vi "App - analyze RUS V6.vi"() -> ()   [LabVIEW 2018] (continued)
"z(0)"=0.0+0.0i, "radius"=0.0}}, "timestamp(min)"=2284.75, "timestamp"=timestamp(3493864906 s since 1904-01-01), "Magn Field(T)"=0.0}, {"temperature"=14.449, "lorentzian"={"A (VHz)"=0.0, "f (Hz)"=0.0, "G (Hz)"=0.0, "phi(rad)"=0.0, "Q"=0.0, "Norm  Ampl"=0.0, "bg (V)"=0.0+0.0i, "4corners"={"z (-pi/2)"=0.0+0.0i, "z(inf)"=0.0+0.0i, "z (pi/2)"=0.0+0.0i, "z center"=0.0+0.0i, "z(0)"=0.0+0.0i, "radius"=0.0}}, "timestamp(min)"=2286.083333335817, "timestamp"=timestamp(3493864986 s since 1904-01-01), "Magn Field(T)"=0.0}, {"temperature"=14.451, "lorentzian"={"A (VHz)"=0.0, "f (Hz)"=0.0, "G (Hz)"=0.0, "phi(rad)"=0.0, "Q"=0.0, "Norm  Ampl"=0.0, "bg (V)"=0.0+0.0i, "4corners"={"z (-pi/2)"=0.0+0.0i, "z(inf)"=0.0+0.0i, "z (pi/2)"=0.0+0.0i, "z center"=0.0+0.0i, "z(0)"=0.0+0.0i, "radius"=0.0}}, "timestamp(min)"=2287.39999999851, "timestamp"=timestamp(3493865065 s since 1904-01-01), "Magn Field(T)"=0.0}, {"temperature"=14.449, "lorentzian"={"A (VHz)"=0.0, "f (Hz)"=0.0, "G (Hz)"=0.0, "phi(rad)"=0.0, "Q"=0.0, "Norm  Ampl"=0.0, "bg (V)"=0.0+0.0i, "4corners"={"z (-pi/2)"=0.0+0.0i, "z(inf)"=0.0+0.0i, "z (pi/2)"=0.0+0.0i, "z center"=0.0+0.0i, "z(0)"=0.0+0.0i, "radius"=0.0}}, "timestamp(min)"=2288.7333333343267, "timestamp"=timestamp(3493865145 s since 1904-01-01), "Magn Field(T)"=0.0}, {"temperature"=14.445, "lorentzian"={"A (VHz)"=0.0, "f (Hz)"=0.0, "G (Hz)"=0.0, "phi(rad)"=0.0, "Q"=0.0, "Norm  Ampl"=0.0, "bg (V)"=0.0+0.0i, "4corners"={"z (-pi/2)"=0.0+0.0i, "z(inf)"=0.0+0.0i, "z (pi/2)"=0.0+0.0i, "z center"=0.0+0.0i, "z(0)"=0.0+0.0i, "radius"=0.0}}, "timestamp(min)"=2290.0500000044703, "timestamp"=timestamp(3493865224 s since 1904-01-01), "Magn Field(T)"=0.0}, {"temperature"=14.447, "lorentzian"={"A (VHz)"=0.0, "f (Hz)"=0.0, "G (Hz)"=0.0, "phi(rad)"=0.0, "Q"=0.0, "Norm  Ampl"=0.0, "bg (V)"=0.0+0.0i, "4corners"={"z (-pi/2)"=0.0+0.0i, "z(inf)"=0.0+0.0i, "z (pi/2)"=0.0+0.0i, "z center"=0.0+0.0i, "z(0)"=0.0+0.0i, "radius"=0.0}}, "timestamp(min)"=2291.3666666671634, "timestamp"=timestamp(3493865303 s since 1904-01-01), "Magn Field(T)"=0.0}, {"temperature"=14.443, "lorentzian"={"A (VHz)"=0.0, "f (Hz)"=0.0, "G (Hz)"=0.0, "phi(rad)"=0.0, "Q"=0.0, "Norm  Ampl"=0.0, "bg (V)"=0.0+0.0i, "4corners"={"z (-pi/2)"=0.0+0.0i, "z(inf)"=0.0+0.0i, "z (pi/2)"=0.0+0.0i, "z center"=0.0+0.0i, "z(0)"=0.0+0.0i, "radius"=0.0}}, "timestamp(min)"=2292.7000000029802, "timestamp"=timestamp(3493865383 s since 1904-01-01), "Magn Field(T)"=0.0}, {"temperature"=14.439, "lorentzian"={"A (VHz)"=0.0, "f (Hz)"=0.0, "G (Hz)"=0.0, "phi(rad)"=0.0, "Q"=0.0, "Norm  Ampl"=0.0, "bg (V)"=0.0+0.0i, "4corners"={"z (-pi/2)"=0.0+0.0i, "z(inf)"=0.0+0.0i, "z (pi/2)"=0.0+0.0i, "z center"=0.0+0.0i, "z(0)"=0.0+0.0i, "radius"=0.0}}, "timestamp(min)"=2294.0166666656733, "timestamp"=timestamp(3493865462 s since 1904-01-01), "Magn Field(T)"=0.0}, {"temperature"=14.439, "lorentzian"={"A (VHz)"=0.0, "f (Hz)"=0.0, "G (Hz)"=0.0, "phi(rad)"=0.0, "Q"=0.0, "Norm  Ampl"=0.0, "bg (V)"=0.0+0.0i, "4corners"={"z (-pi/2)"=0.0+0.0i, "z(inf)"=0.0+0.0i, "z (pi/2)"=0.0+0.0i, "z center"=0.0+0.0i, "z(0)"=0.0+0.0i, "radius"=0.0}}, "timestamp(min)"=2295.333333335817, "timestamp"=timestamp(3493865541 s since 1904-01-01), "Magn Field(T)"=0.0}, {"temperature"=14.439, "lorentzian"={"A (VHz)"=0.0, "f (Hz)"=0.0, "G (Hz)"=0.0, "phi(rad)"=0.0, "Q"=0.0, "Norm  Ampl"=0.0, "bg (V)"=0.0+0.0i, "4corners"={"z (-pi/2)"=0.0+0.0i, "z(inf)"=0.0+0.0i, "z (pi/2)"=0.0+0.0i, "z center"=0.0+0.0i, "z(0)"=0.0+0.0i, "radius"=0.0}}, "timestamp(min)"=2296.666666664183, "timestamp"=timestamp(3493865621 s since 1904-01-01), "Magn Field(T)"=0.0}, {"temperature"=14.439, "lorentzian"={"A (VHz)"=0.0, "f (Hz)"=0.0, "G (Hz)"=0.0, "phi(rad)"=0.0, "Q"=0.0, "Norm  Ampl"=0.0, "bg (V)"=0.0+0.0i, "4corners"={"z (-pi/2)"=0.0+0.0i, "z(inf)"=0.0+0.0i, "z (pi/2)"=0.0+0.0i, "z center"=0.0+0.0i, "z(0)"=0.0+0.0i, "radius"=0.0}}, "timestamp(min)"=2297.9833333343267, "timestamp"=timestamp(3493865700 s since 1904-01-01), "Magn Field(T)"=0.0}, {"temperature"=14.44, "lorentzian"={"A (VHz)"=0.0, "f (Hz)"=0.0, "G (Hz)"=0.0, "phi(rad)"=0.0, "Q"=0.0, "Norm  Ampl"=0.0, "bg (V)"=0.0+0.0i, "4corners"={"z (-pi/2)"=0.0+0.0i, "z(inf)"=0.0+0.0i, "z (pi/2)"=0.0+0.0i, "z center"=0.0+0.0i, "z(0)"=0.0+0.0i, "radius"=0.0}}, "timestamp(min)"=2299.3166666701436, "timestamp"=timestamp(3493865780 s since 1904-01-01), "Magn Field(T)"=0.0}, {"temperature"=14.433, "lorentzian"={"A (VHz)"=0.0, "f (Hz)"=0.0, "G (Hz)"=0.0, "phi(rad)"=0.0, "Q"=0.0, "Norm  Ampl"=0.0, "bg (V)"=0.0+0.0i, "4corners"={"z (-pi/2)"=0.0+0.0i, "z(inf)"=0.0+0.0i, "z (pi/2)"=0.0+0.0i, "z center"=0.0+0.0i, "z(0)"=0.0+0.0i, "radius"=0.0}}, "timestamp(min)"=2300.6333333328366, "timestamp"=timestamp(3493865859 s since 1904-01-01), "Magn Field(T)"=0.0}, {"temperature"=14.434, "lorentzian"={"A (VHz)"=0.0, "f (Hz)"=0.0, "G (Hz)"=0.0, "phi(rad)"=0.0, "Q"=0.0, "Norm  Ampl"=0.0, "bg (V)"=0.0+0.0i, "4corners"={"z (-pi/2)"=0.0+0.0i, "z(inf)"=0.0+0.0i, "z (pi/2)"=0.0+0.0i, "z center"=0.0+0.0i, "z(0)"=0.0+0.0i, "radius"=0.0}}, "timestamp(min)"=2301.9500000029802, "timestamp"=timestamp(3493865938 s since 1904-01-01), "Magn Field(T)"=0.0}, {"temperature"=14.43, "lorentzian"={"A (VHz)"=0.0, "f (Hz)"=0.0, "G (Hz)"=0.0, "phi(rad)"=0.0, "Q"=0.0, "Norm  Ampl"=0.0, "bg (V)"=0.0+0.0i, "4corners"={"z (-pi/2)"=0.0+0.0i, "z(inf)"=0.0+0.0i, "z (pi/2)"=0.0+0.0i, "z center"=0.0+0.0i, "z(0)"=0.0+0.0i, "radius"=0.0}}, "timestamp(min)"=2303.2833333313465, "timestamp"=timestamp(3493866018 s since 1904-01-01), "Magn Field(T)"=0.0}, {"temperature"=14.43, "lorentzian"={"A (VHz)"=0.0, "f (Hz)"=0.0, "G (Hz)"=0.0, "phi(rad)"=0.0, "Q"=0.0, "Norm  Ampl"=0.0, "bg (V)"=0.0+0.0i, "4corners"={"z (-pi/2)"=0.0+0.0i, "z(inf)"=0.0+0.0i, "z (pi/2)"=0.0+0.0i, "z center"=0.0+0.0i, "z(0)"=0.0+0.0i, "radius"=0.0}}, "timestamp(min)"=2304.60000000149, "timestamp"=timestamp(3493866097 s since 1904-01-01), "Magn Field(T)"=0.0}, {"temperature"=14.43, "lorentzian"={"A (VHz)"=0.0, "f (Hz)"=0.0, "G (Hz)"=0.0, "phi(rad)"=0.0, "Q"=0.0, "Norm  Ampl"=0.0, "bg (V)"=0.0+0.0i, "4corners"={"z (-pi/2)"=0.0+0.0i, "z(inf)"=0.0+0.0i, "z (pi/2)"=0.0+0.0i, "z center"=0.0+0.0i, "z(0)"=0.0+0.0i, "radius"=0.0}}, "timestamp(min)"=2305.933333337307, "timestamp"=timestamp(3493866177 s since 1904-01-01), "Magn Field(T)"=0.0}, {"temperature"=14.434, "lorentzian"={"A (VHz)"=0.0, "f (Hz)"=0.0, "G (Hz)"=0.0, "phi(rad)"=0.0, "Q"=0.0, "Norm  Ampl"=0.0, "bg (V)"=0.0+0.0i, "4corners"={"z (-pi/2)"=0.0+0.0i, "z(inf)"=0.0+0.0i, "z (pi/2)"=0.0+0.0i, "z center"=0.0+0.0i, "z(0)"=0.0+0.0i, "radius"=0.0}}, "timestamp(min)"=2307.25, "timestamp"=timestamp(3493866256 s since 1904-01-01), "Magn Field(T)"=0.0}, {"temperature"=14.434, "lorentzian"={"A (VHz)"=0.0, "f (Hz)"=0.0, "G (Hz)"=0.0, "phi(rad)"=0.0, "Q"=0.0, "Norm  Ampl"=0.0, "bg (V)"=0.0+0.0i, "4corners"={"z (-pi/2)"=0.0+0.0i, "z(inf)"=0.0+0.0i, "z (pi/2)"=0.0+0.0i, "z center"=0.0+0.0i, "z(0)"=0.0+0.0i, "radius"=0.0}}, "timestamp(min)"=2308.5666666701436, "timestamp"=timestamp(3493866335 s since 1904-01-01), "Magn Field(T)"=0.0}, {"temperature"=14.431, "lorentzian"={"A (VHz)"=0.0, "f (Hz)"=0.0, "G (Hz)"=0.0, "phi(rad)"=0.0, "Q"=0.0, "Norm  Ampl"=0.0, "bg (V)"=0.0+0.0i, "4corners"={"z (-pi/2)"=0.0+0.0i, "z(inf)"=0.0+0.0i, "z (pi/2)"=0.0+0.0i, "z center"=0.0+0.0i, "z(0)"=0.0+0.0i, "radius"=0.0}}, "timestamp(min)"=2309.89999999851, "timestamp"=timestamp(3493866415 s since 1904-01-01), "Magn Field(T)"=0.0}, {"temperature"=14.429, "lorentzian"={"A (VHz)"=0.0, "f (Hz)"=0.0, "G (Hz)"=0.0, "phi(rad)"=0.0, "Q"=0.0, "Norm  Ampl"=0.0, "bg (V)"=0.0+0.0i, "4corners"={"z (-pi/2)"=0.0+0.0i, "z(inf)"=0.0+0.0i, "z (pi/2)"=0.0+0.0i, "z center"=0.0+0.0i, "z(0)"=0.0+0.0i, "radius"=0.0}}, "timestamp(min)"=2311.2166666686535, "timestamp"=timestamp(3493866494 s since 1904-01-01), "Magn Field(T)"=0.0}, {"temperature"=14.426, "lorentzian"={"A (VHz)"=0.0, "f (Hz)"=0.0, "G (Hz)"=0.0, "phi(rad)"=0.0, "Q"=0.0, "Norm  Ampl"=0.0, "bg (V)"=0.0+0.0i, "4corners"={"z (-pi/2)"=0.0+0.0i, "z(inf)"=0.0+0.0i, "z (pi/2)"=0.0+0.0i, "z center"=0.0+0.0i, "z(0)"=0.0+0.0i, "radius"=0.0}}, "timestamp(min)"=2312.5333333313465, "timestamp"=timestamp(3493866573 s since 1904-01-01), "Magn Field(T)"=0.0}, {"temperature"=14.429, "lorentzian"={"A (VHz)"=0.0, "f (Hz)"=0.0, "G (Hz)"=0.0, "phi(rad)"=0.0, "Q"=0.0, "Norm  Ampl"=0.0, "bg (V)"=0.0+0.0i, "4corners"={"z (-pi/2)"=0.0+0.0i, "z(inf)"=0.0+0.0i, "z (pi/2)"=0.0+0.0i, "z center"=0.0+0.0i, "z(0)"=0.0+0.0i, "radius"=0.0}}, "timestamp(min)"=2313.8666666671634, "timestamp"=timestamp(3493866653 s since 1904-01-01), "Magn Field(T)"=0.0}, {"temperature"=14.429, "lorentzian"={"A (VHz)"=0.0, "f (Hz)"=0.0, "G (Hz)"=0.0, "phi(rad)"=0.0, "Q"=0.0, "Norm  Ampl"=0.0, "bg (V)"=0.0+0.0i, "4corners"={"z (-pi/2)"=0.0+0.0i, "z(inf)"=0.0+0.0i, "z (pi/2)"=0.0+0.0i, "z center"=0.0+0.0i, "z(0)"=0.0+0.0i, "radius"=0.0}}, "timestamp(min)"=2315.183333337307, "timestamp"=timestamp(3493866732 s since 1904-01-01), "Magn Field(T)"=0.0}, {"temperature"=14.425, "lorentzian"={"A (VHz)"=0.0, "f (Hz)"=0.0, "G (Hz)"=0.0, "phi(rad)"=0.0, "Q"=0.0, "Norm  Ampl"=0.0, "bg (V)"=0.0+0.0i, "4corners"={"z (-pi/2)"=0.0+0.0i, "z(inf)"=0.0+0.0i, "z (pi/2)"=0.0+0.0i, "z center"=0.0+0.0i, "z(0)"=0.0+0.0i, "radius"=0.0}}, "timestamp(min)"=2316.5166666656733, "timestamp"=timestamp(3493866812 s since 1904-01-01), "Magn Field(T)"=0.0}, {"temperature"=14.426, "lorentzian"={"A (VHz)"=0.0, "f (Hz)"=0.0, "G (Hz)"=0.0, "phi(rad)"=0.0, "Q"=0.0, "Norm  Ampl"=0.0, "bg (V)"=0.0+0.0i, "4corners"={"z (-pi/2)"=0.0+0.0i, "z(inf)"=0.0+0.0i, "z (pi/2)"=0.0+0.0i, "z center"=0.0+0.0i, "z(0)"=0.0+0.0i, "radius"=0.0}}, "timestamp(min)"=2317.833333335817, "timestamp"=timestamp(3493866891 s since 1904-01-01), "Magn Field(T)"=0.0}, {"temperature"=14.422, "lorentzian"={"A (VHz)"=0.0, "f (Hz)"=0.0, "G (Hz)"=0.0, "phi(rad)"=0.0, "Q"=0.0, "Norm  Ampl"=0.0, "bg (V)"=0.0+0.0i, "4corners"={"z (-pi/2)"=0.0+0.0i, "z(inf)"=0.0+0.0i, "z (pi/2)"=0.0+0.0i, "z center"=0.0+0.0i, "z(0)"=0.0+0.0i, "radius"=0.0}}, "timestamp(min)"=2319.14999999851, "timestamp"=timestamp(3493866970 s since 1904-01-01), "Magn Field(T)"=0.0}, {"temperature"=14.424, "lorentzian"={"A (VHz)"=0.0, "f (Hz)"=0.0, "G (Hz)"=0.0, "phi(rad)"=0.0, "Q"=0.0, "Norm  Ampl"=0.0, "bg (V)"=0.0+0.0i, "4corners"={"z (-pi/2)"=0.0+0.0i, "z(inf)"=0.0+0.0i, "z (pi/2)"=0.0+0.0i, "z center"=0.0+0.0i, "z(0)"=0.0+0.0i, "radius"=0.0}}, "timestamp(min)"=2320.4833333343267, "timestamp"=timestamp(3493867050 s since 1904-01-01), "Magn Field(T)"=0.0}, {"temperature"=14.421, "lorentzian"={"A (VHz)"=0.0, "f (Hz)"=0.0, "G (Hz)"=0.0, "phi(rad)"=0.0, "Q"=0.0, "Norm  Ampl"=0.0, "bg (V)"=0.0+0.0i, "4corners"={"z (-pi/2)"=0.0+0.0i, "z(inf)"=0.0+0.0i, "z (pi/2)"=0.0+0.0i, "z center"=0.0+0.0i, "z(0)"=0.0+0.0i, "radius"=0.0}}, "timestamp(min)"=2321.8000000044703, "timestamp"=timestamp(3493867129 s since 1904-01-01), "Magn Field(T)"=0.0}, {"temperature"=14.418, "lorentzian"={"A (VHz)"=0.0, "f (Hz)"=0.0, "G (Hz)"=0.0, "phi(rad)"=0.0, "Q"=0.0, "Norm  Ampl"=0.0, "bg (V)"=0.0+0.0i, "4corners"={"z (-pi/2)"=0.0+0.0i, "z(inf)"=0.0+0.0i, "z (pi/2)"=0.0+0.0i, "z center"=0.0+0.0i, "z(0)"=0.0+0.0i, "radius"=0.0}}, "timestamp(min)"=2323.1166666671634, "timestamp"=timestamp(3493867208 s since 1904-01-01), "Magn Field(T)"=0.0}, {"temperature"=14.417, "lorentzian"={"A (VHz)"=0.0, "f (Hz)"=0.0, "G (Hz)"=0.0, "phi(rad)"=0.0, "Q"=0.0, "Norm  Ampl"=0.0, "bg (V)"=0.0+0.0i, "4corners"={"z (-pi/2)"=0.0+0.0i, "z(inf)"=0.0+0.0i, "z (pi/2)"=0.0+0.0i, "z center"=0.0+0.0i, "z(0)"=0.0+0.0i, "radius"=0.0}}, "timestamp(min)"=2324.4500000029802, "timestamp"=timestamp(3493867288 s since 1904-01-01), "Magn Field(T)"=0.0}, {"temperature"=14.415, "lorentzian"={"A (VHz)"=0.0, "f (Hz)"=0.0, "G (Hz)"=0.0, "phi(rad)"=0.0, "Q"=0.0, "Norm  Ampl"=0.0, "bg (V)"=0.0+0.0i, "4corners"={"z (-pi/2)"=0.0+0.0i, "z(inf)"=0.0+0.0i, "z (pi/2)"=0.0+0.0i, "z center"=0.0+0.0i, "z(0)"=0.0+0.0i, "radius"=0.0}}, "timestamp(min)"=2325.7666666656733, "timestamp"=timestamp(3493867367 s since 1904-01-01), "Magn Field(T)"=0.0}, {"temperature"=14.413, "lorentzian"={"A (VHz)"=0.0, "f (Hz)"=0.0, "G (Hz)"=0.0, "phi(rad)"=0.0, "Q"=0.0, "Norm  Ampl"=0.0, "bg (V)"=0.0+0.0i, "4corners"={"z (-pi/2)"=0.0+0.0i, "z(inf)"=0.0+0.0i, "z (pi/2)"=0.0+0.0i, "z center"=0.0+0.0i, "z(0)"=0.0+0.0i, "radius"=0.0}}, "timestamp(min)"=2327.10000000149, "timestamp"=timestamp(3493867447 s since 1904-01-01), "Magn Field(T)"=0.0}, {"temperature"=14.414, "lorentzian"={"A (VHz)"=0.0, "f (Hz)"=0.0, "G (Hz)"=0.0, "phi(rad)"=0.0, "Q"=0.0, "Norm  Ampl"=0.0, "bg (V)"=0.0+0.0i, "4corners"={"z (-pi/2)"=0.0+0.0i, "z(inf)"=0.0+0.0i, "z (pi/2)"=0.0+0.0i, "z center"=0.0+0.0i, "z(0)"=0.0+0.0i, "radius"=0.0}}, "timestamp(min)"=2328.416666664183, "timestamp"=timestamp(3493867526 s since 1904-01-01), "Magn Field(T)"=0.0}, {"temperature"=14.412, "lorentzian"={"A (VHz)"=0.0, "f (Hz)"=0.0, "G (Hz)"=0.0, "phi(rad)"=0.0, "Q"=0.0, "Norm  Ampl"=0.0, "bg (V)"=0.0+0.0i, "4corners"={"z (-pi/2)"=0.0+0.0i, "z(inf)"=0.0+0.0i, "z (pi/2)"=0.0+0.0i, "z center"=0.0+0.0i, "z(0)"=0.0+0.0i, "radius"=0.0}}, "timestamp(min)"=2329.7333333343267, "timestamp"=timestamp(3493867605 s since 1904-01-01), "Magn Field(T)"=0.0}, {"temperature"=14.418, "lorentzian"={"A (VHz)"=0.0, "f (Hz)"=0.0, "G (Hz)"=0.0, "phi(rad)"=0.0, "Q"=0.0, "Norm  Ampl"=0.0, "bg (V)"=0.0+0.0i, "4corners"={"z (-pi/2)"=0.0+0.0i, "z(inf)"=0.0+0.0i, "z (pi/2)"=0.0+0.0i, "z center"=0.0+0.0i, "z(0)"=0.0+0.0i, "radius"=0.0}}, "timestamp(min)"=2331.0666666701436, "timestamp"=timestamp(3493867685 s since 1904-01-01), "Magn Field(T)"=0.0}, {"temperature"=14.417, "lorentzian"={"A (VHz)"=0.0, "f (Hz)"=0.0, "G (Hz)"=0.0, "phi(rad)"=0.0, "Q"=0.0, "Norm  Ampl"=0.0, "bg (V)"=0.0+0.0i, "4corners"={"z (-pi/2)"=0.0+0.0i, "z(inf)"=0.0+0.0i, "z (pi/2)"=0.0+0.0i, "z center"=0.0+0.0i, "z(0)"=0.0+0.0i, "radius"=0.0}}, "timestamp(min)"=2332.3833333328366, "timestamp"=timestamp(3493867764 s since 1904-01-01), "Magn Field(T)"=0.0}, {"temperature"=14.412, "lorentzian"={"A (VHz)"=0.0, "f (Hz)"=0.0, "G (Hz)"=0.0, "phi(rad)"=0.0, "Q"=0.0, "Norm  Ampl"=0.0, "bg (V)"=0.0+0.0i, "4corners"={"z (-pi/2)"=0.0+0.0i, "z(inf)"=0.0+0.0i, "z (pi/2)"=0.0+0.0i, "z center"=0.0+0.0i, "z(0)"=0.0+0.0i, "radius"=0.0}}, "timestamp(min)"=2333.7166666686535, "timestamp"=timestamp(3493867844 s since 1904-01-01), "Magn Field(T)"=0.0}, {"temperature"=14.413, "lorentzian"={"A (VHz)"=0.0, "f (Hz)"=0.0, "G (Hz)"=0.0, "phi(rad)"=0.0, "Q"=0.0, "Norm  Ampl"=0.0, "bg (V)"=0.0+0.0i, "4corners"={"z (-pi/2)"=0.0+0.0i, "z(inf)"=0.0+0.0i, "z (pi/2)"=0.0+0.0i, "z center"=0.0+0.0i, "z(0)"=0.0+0.0i, "radius"=0.0}}, "timestamp(min)"=2335.0333333313465, "timestamp"=timestamp(3493867923 s since 1904-01-01), "Magn Field(T)"=0.0}, {"temperature"=14.41, "lorentzian"={"A (VHz)"=0.0, "f (Hz)"=0.0, "G (Hz)"=0.0, "phi(rad)"=0.0, "Q"=0.0, "Norm  Ampl"=0.0, "bg (V)"=0.0+0.0i, "4corners"={"z (-pi/2)"=0.0+0.0i, "z(inf)"=0.0+0.0i, "z (pi/2)"=0.0+0.0i, "z center"=0.0+0.0i, "z(0)"=0.0+0.0i, "radius"=0.0}}, "timestamp(min)"=2336.35000000149, "timestamp"=timestamp(3493868002 s since 1904-01-01), "Magn Field(T)"=0.0}, {"temperature"=14.414, "lorentzian"={"A (VHz)"=0.0, "f (Hz)"=0.0, "G (Hz)"=0.0, "phi(rad)"=0.0, "Q"=0.0, "Norm  Ampl"=0.0, "bg (V)"=0.0+0.0i, "4corners"={"z (-pi/2)"=0.0+0.0i, "z(inf)"=0.0+0.0i, "z (pi/2)"=0.0+0.0i, "z center"=0.0+0.0i, "z(0)"=0.0+0.0i, "radius"=0.0}}, "timestamp(min)"=2337.683333337307, "timestamp"=timestamp(3493868082 s since 1904-01-01), "Magn Field(T)"=0.0}, {"temperature"=14.408, "lorentzian"={"A (VHz)"=0.0, "f (Hz)"=0.0, "G (Hz)"=0.0, "phi(rad)"=0.0, "Q"=0.0, "Norm  Ampl"=0.0, "bg (V)"=0.0+0.0i, "4corners"={"z (-pi/2)"=0.0+0.0i, "z(inf)"=0.0+0.0i, "z (pi/2)"=0.0+0.0i, "z center"=0.0+0.0i, "z(0)"=0.0+0.0i, "radius"=0.0}}, "timestamp(min)"=2339.0, "timestamp"=timestamp(3493868161 s since 1904-01-01), "Magn Field(T)"=0.0}, {"temperature"=14.407, "lorentzian"={"A (VHz)"=0.0, "f (Hz)"=0.0, "G (Hz)"=0.0, "phi(rad)"=0.0, "Q"=0.0, "Norm  Ampl"=0.0, "bg (V)"=0.0+0.0i, "4corners"={"z (-pi/2)"=0.0+0.0i, "z(inf)"=0.0+0.0i, "z (pi/2)"=0.0+0.0i, "z center"=0.0+0.0i, "z(0)"=0.0+0.0i, "radius"=0.0}}, "timestamp(min)"=2340.3166666701436, "timestamp"=timestamp(3493868240 s since 1904-01-01), "Magn Field(T)"=0.0}, {"temperature"=14.406, "lorentzian"={"A (VHz)"=0.0, "f (Hz)"=0.0, "G (Hz)"=0.0, "phi(rad)"=0.0, "Q"=0.0, "Norm  Ampl"=0.0, "bg (V)"=0.0+0.0i, "4corners"={"z (-pi/2)"=0.0+0.0i, "z(inf)"=0.0+0.0i, "z (pi/2)"=0.0+0.0i, "z center"=0.0+0.0i, "z(0)"=0.0+0.0i, "radius"=0.0}}, "timestamp(min)"=2341.64999999851, "timestamp"=timestamp(3493868320 s since 1904-01-01), "Magn Field(T)"=0.0}, {"temperature"=14.402, "lorentzian"={"A (VHz)"=0.0, "f (Hz)"=0.0, "G (Hz)"=0.0, "phi(rad)"=0.0, "Q"=0.0, "Norm  Ampl"=0.0, "bg (V)"=0.0+0.0i, "4corners"={"z (-pi/2)"=0.0+0.0i, "z(inf)"=0.0+0.0i, "z (pi/2)"=0.0+0.0i, "z center"=0.0+0.0i, "z(0)"=0.0+0.0i, "radius"=0.0}}, "timestamp(min)"=2342.9666666686535, "timestamp"=timestamp(3493868399 s since 1904-01-01), "Magn Field(T)"=0.0}, {"temperature"=14.4, "lorentzian"={"A (VHz)"=0.0, "f (Hz)"=0.0, "G (Hz)"=0.0, "phi(rad)"=0.0, "Q"=0.0, "Norm  Ampl"=0.0, "bg (V)"=0.0+0.0i, "4corners"={"z (-pi/2)"=0.0+0.0i, "z(inf)"=0.0+0.0i, "z (pi/2)"=0.0+0.0i, "z center"=0.0+0.0i, "z(0)"=0.0+0.0i, "radius"=0.0}}, "timestamp(min)"=2344.3000000044703, "timestamp"=timestamp(3493868479 s since 1904-01-01), "Magn Field(T)"=0.0}, {"temperature"=14.396, "lorentzian"={"A (VHz)"=0.0, "f (Hz)"=0.0, "G (Hz)"=0.0, "phi(rad)"=0.0, "Q"=0.0, "Norm  Ampl"=0.0, "bg (V)"=0.0+0.0i, "4corners"={"z (-pi/2)"=0.0+0.0i, "z(inf)"=0.0+0.0i, "z (pi/2)"=0.0+0.0i, "z center"=0.0+0.0i, "z(0)"=0.0+0.0i, "radius"=0.0}}, "timestamp(min)"=2345.6166666671634, "timestamp"=timestamp(3493868558 s since 1904-01-01), "Magn Field(T)"=0.0}, {"temperature"=14.394, "lorentzian"={"A (VHz)"=0.0, "f (Hz)"=0.0, "G (Hz)"=0.0, "phi(rad)"=0.0, "Q"=0.0, "Norm  Ampl"=0.0, "bg (V)"=0.0+0.0i, "4corners"={"z (-pi/2)"=0.0+0.0i, "z(inf)"=0.0+0.0i, "z (pi/2)"=0.0+0.0i, "z center"=0.0+0.0i, "z(0)"=0.0+0.0i, "radius"=0.0}}, "timestamp(min)"=2346.933333337307, "timestamp"=timestamp(3493868637 s since 1904-01-01), "Magn Field(T)"=0.0}, {"temperature"=14.393, "lorentzian"={"A (VHz)"=0.0, "f (Hz)"=0.0, "G (Hz)"=0.0, "phi(rad)"=0.0, "Q"=0.0, "Norm  Ampl"=0.0, "bg (V)"=0.0+0.0i, "4corners"={"z (-pi/2)"=0.0+0.0i, "z(inf)"=0.0+0.0i, "z (pi/2)"=0.0+0.0i, "z center"=0.0+0.0i, "z(0)"=0.0+0.0i, "radius"=0.0}}, "timestamp(min)"=2348.2666666656733, "timestamp"=timestamp(3493868717 s since 1904-01-01), "Magn Field(T)"=0.0}, {"temperature"=14.39, "lorentzian"={"A (VHz)"=0.0, "f (Hz)"=0.0, "G (Hz)"=0.0, "phi(rad)"=0.0, "Q"=0.0, "Norm  Ampl"=0.0, "bg (V)"=0.0+0.0i, "4corners"={"z (-pi/2)"=0.0+0.0i, "z(inf)"=0.0+0.0i, "z (pi/2)"=0.0+0.0i, "z center"=0.0+0.0i, "z(0)"=0.0+0.0i, "radius"=0.0}}, "timestamp(min)"=2349.583333335817, "timestamp"=timestamp(3493868796 s since 1904-01-01), "Magn Field(T)"=0.0}, {"temperature"=14.387, "lorentzian"={"A (VHz)"=0.0, "f (Hz)"=0.0, "G (Hz)"=0.0, "phi(rad)"=0.0, "Q"=0.0, "Norm  Ampl"=0.0, "bg (V)"=0.0+0.0i, "4corners"={"z (-pi/2)"=0.0+0.0i, "z(inf)"=0.0+0.0i, "z (pi/2)"=0.0+0.0i, "z center"=0.0+0.0i, "z(0)"=0.0+0.0i, "radius"=0.0}}, "timestamp(min)"=2350.916666664183, "timestamp"=timestamp(3493868876 s since 1904-01-01), "Magn Field(T)"=0.0}, {"temperature"=14.39, "lorentzian"={"A (VHz)"=0.0, "f (Hz)"=0.0, "G (Hz)"=0.0, "phi(rad)"=0.0, "Q"=0.0, "Norm  Ampl"=0.0, "bg (V)"=0.0+0.0i, "4corners"={"z (-pi/2)"=0.0+0.0i, "z(inf)"=0.0+0.0i, "z (pi/2)"=0.0+0.0i, "z center"=0.0+0.0i, "z(0)"=0.0+0.0i, "radius"=0.0}}, "timestamp(min)"=2352.2333333343267, "timestamp"=timestamp(3493868955 s since 1904-01-01), "Magn Field(T)"=0.0}, {"temperature"=14.385, "lorentzian"={"A (VHz)"=0.0, "f (Hz)"=0.0, "G (Hz)"=0.0, "phi(rad)"=0.0, "Q"=0.0, "Norm  Ampl"=0.0, "bg (V)"=0.0+0.0i, "4corners"={"z (-pi/2)"=0.0+0.0i, "z(inf)"=0.0+0.0i, "z (pi/2)"=0.0+0.0i, "z center"=0.0+0.0i, "z(0)"=0.0+0.0i, "radius"=0.0}}, "timestamp(min)"=2353.5500000044703, "timestamp"=timestamp(3493869034 s since 1904-01-01), "Magn Field(T)"=0.0}, {"temperature"=14.384, "lorentzian"={"A (VHz)"=0.0, "f (Hz)"=0.0, "G (Hz)"=0.0, "phi(rad)"=0.0, "Q"=0.0, "Norm  Ampl"=0.0, "bg (V)"=0.0+0.0i, "4corners"={"z (-pi/2)"=0.0+0.0i, "z(inf)"=0.0+0.0i, "z (pi/2)"=0.0+0.0i, "z center"=0.0+0.0i, "z(0)"=0.0+0.0i, "radius"=0.0}}, "timestamp(min)"=2354.8833333328366, "timestamp"=timestamp(3493869114 s since 1904-01-01), "Magn Field(T)"=0.0}, {"temperature"=14.387, "lorentzian"={"A (VHz)"=0.0, "f (Hz)"=0.0, "G (Hz)"=0.0, "phi(rad)"=0.0, "Q"=0.0, "Norm  Ampl"=0.0, "bg (V)"=0.0+0.0i, "4corners"={"z (-pi/2)"=0.0+0.0i, "z(inf)"=0.0+0.0i, "z (pi/2)"=0.0+0.0i, "z center"=0.0+0.0i, "z(0)"=0.0+0.0i, "radius"=0.0}}, "timestamp(min)"=2356.2000000029802, "timestamp"=timestamp(3493869193 s since 1904-01-01), "Magn Field(T)"=0.0}, {"temperature"=14.388, "lorentzian"={"A (VHz)"=0.0, "f (Hz)"=0.0, "G (Hz)"=0.0, "phi(rad)"=0.0, "Q"=0.0, "Norm  Ampl"=0.0, "bg (V)"=0.0+0.0i, "4corners"={"z (-pi/2)"=0.0+0.0i, "z(inf)"=0.0+0.0i, "z (pi/2)"=0.0+0.0i, "z center"=0.0+0.0i, "z(0)"=0.0+0.0i, "radius"=0.0}}, "timestamp(min)"=2357.5166666656733, "timestamp"=timestamp(3493869272 s since 1904-01-01), "Magn Field(T)"=0.0}, {"temperature"=14.382, "lorentzian"={"A (VHz)"=0.0, "f (Hz)"=0.0, "G (Hz)"=0.0, "phi(rad)"=0.0, "Q"=0.0, "Norm  Ampl"=0.0, "bg (V)"=0.0+0.0i, "4corners"={"z (-pi/2)"=0.0+0.0i, "z(inf)"=0.0+0.0i, "z (pi/2)"=0.0+0.0i, "z center"=0.0+0.0i, "z(0)"=0.0+0.0i, "radius"=0.0}}, "timestamp(min)"=2358.85000000149, "timestamp"=timestamp(3493869352 s since 1904-01-01), "Magn Field(T)"=0.0}, {"temperature"=14.384, "lorentzian"={"A (VHz)"=0.0, "f (Hz)"=0.0, "G (Hz)"=0.0, "phi(rad)"=0.0, "Q"=0.0, "Norm  Ampl"=0.0, "bg (V)"=0.0+0.0i, "4corners"={"z (-pi/2)"=0.0+0.0i, "z(inf)"=0.0+0.0i, "z (pi/2)"=0.0+0.0i, "z center"=0.0+0.0i, "z(0)"=0.0+0.0i, "radius"=0.0}}, "timestamp(min)"=2360.166666664183, "timestamp"=timestamp(3493869431 s since 1904-01-01), "Magn Field(T)"=0.0}, {"temperature"=14.381, "lorentzian"={"A (VHz)"=0.0, "f (Hz)"=0.0, "G (Hz)"=0.0, "phi(rad)"=0.0, "Q"=0.0, "Norm  Ampl"=0.0, "bg (V)"=0.0+0.0i, "4corners"={"z (-pi/2)"=0.0+0.0i, "z(inf)"=0.0+0.0i, "z (pi/2)"=0.0+0.0i, "z center"=0.0+0.0i, "z(0)"=0.0+0.0i, "radius"=0.0}}, "timestamp(min)"=2361.5, "timestamp"=timestamp(3493869511 s since 1904-01-01), "Magn Field(T)"=0.0}, {"temperature"=14.381, "lorentzian"={"A (VHz)"=0.0, "f (Hz)"=0.0, "G (Hz)"=0.0, "phi(rad)"=0.0, "Q"=0.0, "Norm  Ampl"=0.0, "bg (V)"=0.0+0.0i, "4corners"={"z (-pi/2)"=0.0+0.0i, "z(inf)"=0.0+0.0i, "z (pi/2)"=0.0+0.0i, "z center"=0.0+0.0i, "z(0)"=0.0+0.0i, "radius"=0.0}}, "timestamp(min)"=2362.8166666701436, "timestamp"=timestamp(3493869590 s since 1904-01-01), "Magn Field(T)"=0.0}, {"temperature"=14.376, "lorentzian"={"A (VHz)"=0.0, "f (Hz)"=0.0, "G (Hz)"=0.0, "phi(rad)"=0.0, "Q"=0.0, "Norm  Ampl"=0.0, "bg (V)"=0.0+0.0i, "4corners"={"z (-pi/2)"=0.0+0.0i, "z(inf)"=0.0+0.0i, "z (pi/2)"=0.0+0.0i, "z center"=0.0+0.0i, "z(0)"=0.0+0.0i, "radius"=0.0}}, "timestamp(min)"=2364.1333333328366, "timestamp"=timestamp(3493869669 s since 1904-01-01), "Magn Field(T)"=0.0}, {"temperature"=14.375, "lorentzian"={"A (VHz)"=0.0, "f (Hz)"=0.0, "G (Hz)"=0.0, "phi(rad)"=0.0, "Q"=0.0, "Norm  Ampl"=0.0, "bg (V)"=0.0+0.0i, "4corners"={"z (-pi/2)"=0.0+0.0i, "z(inf)"=0.0+0.0i, "z (pi/2)"=0.0+0.0i, "z center"=0.0+0.0i, "z(0)"=0.0+0.0i, "radius"=0.0}}, "timestamp(min)"=2365.4666666686535, "timestamp"=timestamp(3493869749 s since 1904-01-01), "Magn Field(T)"=0.0}, {"temperature"=14.371, "lorentzian"={"A (VHz)"=0.0, "f (Hz)"=0.0, "G (Hz)"=0.0, "phi(rad)"=0.0, "Q"=0.0, "Norm  Ampl"=0.0, "bg (V)"=0.0+0.0i, "4corners"={"z (-pi/2)"=0.0+0.0i, "z(inf)"=0.0+0.0i, "z (pi/2)"=0.0+0.0i, "z center"=0.0+0.0i, "z(0)"=0.0+0.0i, "radius"=0.0}}, "timestamp(min)"=2366.7833333313465, "timestamp"=timestamp(3493869828 s since 1904-01-01), "Magn Field(T)"=0.0}, {"temperature"=14.371, "lorentzian"={"A (VHz)"=0.0, "f (Hz)"=0.0, "G (Hz)"=0.0, "phi(rad)"=0.0, "Q"=0.0, "Norm  Ampl"=0.0, "bg (V)"=0.0+0.0i, "4corners"={"z (-pi/2)"=0.0+0.0i, "z(inf)"=0.0+0.0i, "z (pi/2)"=0.0+0.0i, "z center"=0.0+0.0i, "z(0)"=0.0+0.0i, "radius"=0.0}}, "timestamp(min)"=2368.10000000149, "timestamp"=timestamp(3493869907 s since 1904-01-01), "Magn Field(T)"=0.0}, {"temperature"=14.369, "lorentzian"={"A (VHz)"=0.0, "f (Hz)"=0.0, "G (Hz)"=0.0, "phi(rad)"=0.0, "Q"=0.0, "Norm  Ampl"=0.0, "bg (V)"=0.0+0.0i, "4corners"={"z (-pi/2)"=0.0+0.0i, "z(inf)"=0.0+0.0i, "z (pi/2)"=0.0+0.0i, "z center"=0.0+0.0i, "z(0)"=0.0+0.0i, "radius"=0.0}}, "timestamp(min)"=2369.433333337307, "timestamp"=timestamp(3493869987 s since 1904-01-01), "Magn Field(T)"=0.0}, {"temperature"=14.369, "lorentzian"={"A (VHz)"=0.0, "f (Hz)"=0.0, "G (Hz)"=0.0, "phi(rad)"=0.0, "Q"=0.0, "Norm  Ampl"=0.0, "bg (V)"=0.0+0.0i, "4corners"={"z (-pi/2)"=0.0+0.0i, "z(inf)"=0.0+0.0i, "z (pi/2)"=0.0+0.0i, "z center"=0.0+0.0i, "z(0)"=0.0+0.0i, "radius"=0.0}}, "timestamp(min)"=2370.75, "timestamp"=timestamp(3493870066 s since 1904-01-01), "Magn Field(T)"=0.0}, {"temperature"=14.373, "lorentzian"={"A (VHz)"=0.0, "f (Hz)"=0.0, "G (Hz)"=0.0, "phi(rad)"=0.0, "Q"=0.0, "Norm  Ampl"=0.0, "bg (V)"=0.0+0.0i, "4corners"={"z (-pi/2)"=0.0+0.0i, "z(inf)"=0.0+0.0i, "z (pi/2)"=0.0+0.0i, "z center"=0.0+0.0i, "z(0)"=0.0+0.0i, "radius"=0.0}}, "timestamp(min)"=2372.083333335817, "timestamp"=timestamp(3493870146 s since 1904-01-01), "Magn Field(T)"=0.0}, {"temperature"=14.37, "lorentzian"={"A (VHz)"=0.0, "f (Hz)"=0.0, "G (Hz)"=0.0, "phi(rad)"=0.0, "Q"=0.0, "Norm  Ampl"=0.0, "bg (V)"=0.0+0.0i, "4corners"={"z (-pi/2)"=0.0+0.0i, "z(inf)"=0.0+0.0i, "z (pi/2)"=0.0+0.0i, "z center"=0.0+0.0i, "z(0)"=0.0+0.0i, "radius"=0.0}}, "timestamp(min)"=2373.39999999851, "timestamp"=timestamp(3493870225 s since 1904-01-01), "Magn Field(T)"=0.0}, {"temperature"=14.368, "lorentzian"={"A (VHz)"=0.0, "f (Hz)"=0.0, "G (Hz)"=0.0, "phi(rad)"=0.0, "Q"=0.0, "Norm  Ampl"=0.0, "bg (V)"=0.0+0.0i, "4corners"={"z (-pi/2)"=0.0+0.0i, "z(inf)"=0.0+0.0i, "z (pi/2)"=0.0+0.0i, "z center"=0.0+0.0i, "z(0)"=0.0+0.0i, "radius"=0.0}}, "timestamp(min)"=2374.7166666686535, "timestamp"=timestamp(3493870304 s since 1904-01-01), "Magn Field(T)"=0.0}, {"temperature"=14.366, "lorentzian"={"A (VHz)"=0.0, "f (Hz)"=0.0, "G (Hz)"=0.0, "phi(rad)"=0.0, "Q"=0.0, "Norm  Ampl"=0.0, "bg (V)"=0.0+0.0i, "4corners"={"z (-pi/2)"=0.0+0.0i, "z(inf)"=0.0+0.0i, "z (pi/2)"=0.0+0.0i, "z center"=0.0+0.0i, "z(0)"=0.0+0.0i, "radius"=0.0}}, "timestamp(min)"=2376.0500000044703, "timestamp"=timestamp(3493870384 s since 1904-01-01), "Magn Field(T)"=0.0}, {"temperature"=14.363, "lorentzian"={"A (VHz)"=0.0, "f (Hz)"=0.0, "G (Hz)"=0.0, "phi(rad)"=0.0, "Q"=0.0, "Norm  Ampl"=0.0, "bg (V)"=0.0+0.0i, "4corners"={"z (-pi/2)"=0.0+0.0i, "z(inf)"=0.0+0.0i, "z (pi/2)"=0.0+0.0i, "z center"=0.0+0.0i, "z(0)"=0.0+0.0i, "radius"=0.0}}, "timestamp(min)"=2377.3666666671634, "timestamp"=timestamp(3493870463 s since 1904-01-01), "Magn Field(T)"=0.0}, {"temperature"=14.364, "lorentzian"={"A (VHz)"=0.0, "f (Hz)"=0.0, "G (Hz)"=0.0, "phi(rad)"=0.0, "Q"=0.0, "Norm  Ampl"=0.0, "bg (V)"=0.0+0.0i, "4corners"={"z (-pi/2)"=0.0+0.0i, "z(inf)"=0.0+0.0i, "z (pi/2)"=0.0+0.0i, "z center"=0.0+0.0i, "z(0)"=0.0+0.0i, "radius"=0.0}}, "timestamp(min)"=2378.7000000029802, "timestamp"=timestamp(3493870543 s since 1904-01-01), "Magn Field(T)"=0.0}, {"temperature"=14.367, "lorentzian"={"A (VHz)"=0.0, "f (Hz)"=0.0, "G (Hz)"=0.0, "phi(rad)"=0.0, "Q"=0.0, "Norm  Ampl"=0.0, "bg (V)"=0.0+0.0i, "4corners"={"z (-pi/2)"=0.0+0.0i, "z(inf)"=0.0+0.0i, "z (pi/2)"=0.0+0.0i, "z center"=0.0+0.0i, "z(0)"=0.0+0.0i, "radius"=0.0}}, "timestamp(min)"=2380.0166666656733, "timestamp"=timestamp(3493870622 s since 1904-01-01), "Magn Field(T)"=0.0}, {"temperature"=14.363, "lorentzian"={"A (VHz)"=0.0, "f (Hz)"=0.0, "G (Hz)"=0.0, "phi(rad)"=0.0, "Q"=0.0, "Norm  Ampl"=0.0, "bg (V)"=0.0+0.0i, "4corners"={"z (-pi/2)"=0.0+0.0i, "z(inf)"=0.0+0.0i, "z (pi/2)"=0.0+0.0i, "z center"=0.0+0.0i, "z(0)"=0.0+0.0i, "radius"=0.0}}, "timestamp(min)"=2381.333333335817, "timestamp"=timestamp(3493870701 s since 1904-01-01), "Magn Field(T)"=0.0}, {"temperature"=14.363, "lorentzian"={"A (VHz)"=0.0, "f (Hz)"=0.0, "G (Hz)"=0.0, "phi(rad)"=0.0, "Q"=0.0, "Norm  Ampl"=0.0, "bg (V)"=0.0+0.0i, "4corners"={"z (-pi/2)"=0.0+0.0i, "z(inf)"=0.0+0.0i, "z (pi/2)"=0.0+0.0i, "z center"=0.0+0.0i, "z(0)"=0.0+0.0i, "radius"=0.0}}, "timestamp(min)"=2382.666666664183, "timestamp"=timestamp(3493870781 s since 1904-01-01), "Magn Field(T)"=0.0}, {"temperature"=14.363, "lorentzian"={"A (VHz)"=0.0, "f (Hz)"=0.0, "G (Hz)"=0.0, "phi(rad)"=0.0, "Q"=0.0, "Norm  Ampl"=0.0, "bg (V)"=0.0+0.0i, "4corners"={"z (-pi/2)"=0.0+0.0i, "z(inf)"=0.0+0.0i, "z (pi/2)"=0.0+0.0i, "z center"=0.0+0.0i, "z(0)"=0.0+0.0i, "radius"=0.0}}, "timestamp(min)"=2383.9833333343267, "timestamp"=timestamp(3493870860 s since 1904-01-01), "Magn Field(T)"=0.0}, {"temperature"=14.36, "lorentzian"={"A (VHz)"=0.0, "f (Hz)"=0.0, "G (Hz)"=0.0, "phi(rad)"=0.0, "Q"=0.0, "Norm  Ampl"=0.0, "bg (V)"=0.0+0.0i, "4corners"={"z (-pi/2)"=0.0+0.0i, "z(inf)"=0.0+0.0i, "z (pi/2)"=0.0+0.0i, "z center"=0.0+0.0i, "z(0)"=0.0+0.0i, "radius"=0.0}}, "timestamp(min)"=2385.3000000044703, "timestamp"=timestamp(3493870939 s since 1904-01-01), "Magn Field(T)"=0.0}, {"temperature"=14.361, "lorentzian"={"A (VHz)"=0.0, "f (Hz)"=0.0, "G (Hz)"=0.0, "phi(rad)"=0.0, "Q"=0.0, "Norm  Ampl"=0.0, "bg (V)"=0.0+0.0i, "4corners"={"z (-pi/2)"=0.0+0.0i, "z(inf)"=0.0+0.0i, "z (pi/2)"=0.0+0.0i, "z center"=0.0+0.0i, "z(0)"=0.0+0.0i, "radius"=0.0}}, "timestamp(min)"=2386.6333333328366, "timestamp"=timestamp(3493871019 s since 1904-01-01), "Magn Field(T)"=0.0}, {"temperature"=14.361, "lorentzian"={"A (VHz)"=0.0, "f (Hz)"=0.0, "G (Hz)"=0.0, "phi(rad)"=0.0, "Q"=0.0, "Norm  Ampl"=0.0, "bg (V)"=0.0+0.0i, "4corners"={"z (-pi/2)"=0.0+0.0i, "z(inf)"=0.0+0.0i, "z (pi/2)"=0.0+0.0i, "z center"=0.0+0.0i, "z(0)"=0.0+0.0i, "radius"=0.0}}, "timestamp(min)"=2387.9500000029802, "timestamp"=timestamp(3493871098 s since 1904-01-01), "Magn Field(T)"=0.0}, {"temperature"=14.357, "lorentzian"={"A (VHz)"=0.0, "f (Hz)"=0.0, "G (Hz)"=0.0, "phi(rad)"=0.0, "Q"=0.0, "Norm  Ampl"=0.0, "bg (V)"=0.0+0.0i, "4corners"={"z (-pi/2)"=0.0+0.0i, "z(inf)"=0.0+0.0i, "z (pi/2)"=0.0+0.0i, "z center"=0.0+0.0i, "z(0)"=0.0+0.0i, "radius"=0.0}}, "timestamp(min)"=2389.2833333313465, "timestamp"=timestamp(3493871178 s since 1904-01-01), "Magn Field(T)"=0.0}, {"temperature"=14.357, "lorentzian"={"A (VHz)"=0.0, "f (Hz)"=0.0, "G (Hz)"=0.0, "phi(rad)"=0.0, "Q"=0.0, "Norm  Ampl"=0.0, "bg (V)"=0.0+0.0i, "4corners"={"z (-pi/2)"=0.0+0.0i, "z(inf)"=0.0+0.0i, "z (pi/2)"=0.0+0.0i, "z center"=0.0+0.0i, "z(0)"=0.0+0.0i, "radius"=0.0}}, "timestamp(min)"=2390.60000000149, "timestamp"=timestamp(3493871257 s since 1904-01-01), "Magn Field(T)"=0.0}, {"temperature"=14.355, "lorentzian"={"A (VHz)"=0.0, "f (Hz)"=0.0, "G (Hz)"=0.0, "phi(rad)"=0.0, "Q"=0.0, "Norm  Ampl"=0.0, "bg (V)"=0.0+0.0i, "4corners"={"z (-pi/2)"=0.0+0.0i, "z(inf)"=0.0+0.0i, "z (pi/2)"=0.0+0.0i, "z center"=0.0+0.0i, "z(0)"=0.0+0.0i, "radius"=0.0}}, "timestamp(min)"=2391.916666664183, "timestamp"=timestamp(3493871336 s since 1904-01-01), "Magn Field(T)"=0.0}, {"temperature"=14.354, "lorentzian"={"A (VHz)"=0.0, "f (Hz)"=0.0, "G (Hz)"=0.0, "phi(rad)"=0.0, "Q"=0.0, "Norm  Ampl"=0.0, "bg (V)"=0.0+0.0i, "4corners"={"z (-pi/2)"=0.0+0.0i, "z(inf)"=0.0+0.0i, "z (pi/2)"=0.0+0.0i, "z center"=0.0+0.0i, "z(0)"=0.0+0.0i, "radius"=0.0}}, "timestamp(min)"=2393.25, "timestamp"=timestamp(3493871416 s since 1904-01-01), "Magn Field(T)"=0.0}, {"temperature"=14.354, "lorentzian"={"A (VHz)"=0.0, "f (Hz)"=0.0, "G (Hz)"=0.0, "phi(rad)"=0.0, "Q"=0.0, "Norm  Ampl"=0.0, "bg (V)"=0.0+0.0i, "4corners"={"z (-pi/2)"=0.0+0.0i, "z(inf)"=0.0+0.0i, "z (pi/2)"=0.0+0.0i, "z center"=0.0+0.0i, "z(0)"=0.0+0.0i, "radius"=0.0}}, "timestamp(min)"=2394.5666666701436, "timestamp"=timestamp(3493871495 s since 1904-01-01), "Magn Field(T)"=0.0}, {"temperature"=14.352, "lorentzian"={"A (VHz)"=0.0, "f (Hz)"=0.0, "G (Hz)"=0.0, "phi(rad)"=0.0, "Q"=0.0, "Norm  Ampl"=0.0, "bg (V)"=0.0+0.0i, "4corners"={"z (-pi/2)"=0.0+0.0i, "z(inf)"=0.0+0.0i, "z (pi/2)"=0.0+0.0i, "z center"=0.0+0.0i, "z(0)"=0.0+0.0i, "radius"=0.0}}, "timestamp(min)"=2395.8833333328366, "timestamp"=timestamp(3493871574 s since 1904-01-01), "Magn Field(T)"=0.0}, {"temperature"=14.349, "lorentzian"={"A (VHz)"=0.0, "f (Hz)"=0.0, "G (Hz)"=0.0, "phi(rad)"=0.0, "Q"=0.0, "Norm  Ampl"=0.0, "bg (V)"=0.0+0.0i, "4corners"={"z (-pi/2)"=0.0+0.0i, "z(inf)"=0.0+0.0i, "z (pi/2)"=0.0+0.0i, "z center"=0.0+0.0i, "z(0)"=0.0+0.0i, "radius"=0.0}}, "timestamp(min)"=2397.2166666686535, "timestamp"=timestamp(3493871654 s since 1904-01-01), "Magn Field(T)"=0.0}, {"temperature"=14.353, "lorentzian"={"A (VHz)"=0.0, "f (Hz)"=0.0, "G (Hz)"=0.0, "phi(rad)"=0.0, "Q"=0.0, "Norm  Ampl"=0.0, "bg (V)"=0.0+0.0i, "4corners"={"z (-pi/2)"=0.0+0.0i, "z(inf)"=0.0+0.0i, "z (pi/2)"=0.0+0.0i, "z center"=0.0+0.0i, "z(0)"=0.0+0.0i, "radius"=0.0}}, "timestamp(min)"=2398.5333333313465, "timestamp"=timestamp(3493871733 s since 1904-01-01), "Magn Field(T)"=0.0}, {"temperature"=14.35, "lorentzian"={"A (VHz)"=0.0, "f (Hz)"=0.0, "G (Hz)"=0.0, "phi(rad)"=0.0, "Q"=0.0, "Norm  Ampl"=0.0, "bg (V)"=0.0+0.0i, "4corners"={"z (-pi/2)"=0.0+0.0i, "z(inf)"=0.0+0.0i, "z (pi/2)"=0.0+0.0i, "z center"=0.0+0.0i, "z(0)"=0.0+0.0i, "radius"=0.0}}, "timestamp(min)"=2399.8666666671634, "timestamp"=timestamp(3493871813 s since 1904-01-01), "Magn Field(T)"=0.0}, {"temperature"=14.351, "lorentzian"={"A (VHz)"=0.0, "f (Hz)"=0.0, "G (Hz)"=0.0, "phi(rad)"=0.0, "Q"=0.0, "Norm  Ampl"=0.0, "bg (V)"=0.0+0.0i, "4corners"={"z (-pi/2)"=0.0+0.0i, "z(inf)"=0.0+0.0i, "z (pi/2)"=0.0+0.0i, "z center"=0.0+0.0i, "z(0)"=0.0+0.0i, "radius"=0.0}}, "timestamp(min)"=2401.183333337307, "timestamp"=timestamp(3493871892 s since 1904-01-01), "Magn Field(T)"=0.0}, {"temperature"=14.351, "lorentzian"={"A (VHz)"=0.0, "f (Hz)"=0.0, "G (Hz)"=0.0, "phi(rad)"=0.0, "Q"=0.0, "Norm  Ampl"=0.0, "bg (V)"=0.0+0.0i, "4corners"={"z (-pi/2)"=0.0+0.0i, "z(inf)"=0.0+0.0i, "z (pi/2)"=0.0+0.0i, "z center"=0.0+0.0i, "z(0)"=0.0+0.0i, "radius"=0.0}}, "timestamp(min)"=2402.5, "timestamp"=timestamp(3493871971 s since 1904-01-01), "Magn Field(T)"=0.0}, {"temperature"=14.353, "lorentzian"={"A (VHz)"=0.0, "f (Hz)"=0.0, "G (Hz)"=0.0, "phi(rad)"=0.0, "Q"=0.0, "Norm  Ampl"=0.0, "bg (V)"=0.0+0.0i, "4corners"={"z (-pi/2)"=0.0+0.0i, "z(inf)"=0.0+0.0i, "z (pi/2)"=0.0+0.0i, "z center"=0.0+0.0i, "z(0)"=0.0+0.0i, "radius"=0.0}}, "timestamp(min)"=2403.833333335817, "timestamp"=timestamp(3493872051 s since 1904-01-01), "Magn Field(T)"=0.0}, {"temperature"=14.352, "lorentzian"={"A (VHz)"=0.0, "f (Hz)"=0.0, "G (Hz)"=0.0, "phi(rad)"=0.0, "Q"=0.0, "Norm  Ampl"=0.0, "bg (V)"=0.0+0.0i, "4corners"={"z (-pi/2)"=0.0+0.0i, "z(inf)"=0.0+0.0i, "z (pi/2)"=0.0+0.0i, "z center"=0.0+0.0i, "z(0)"=0.0+0.0i, "radius"=0.0}}, "timestamp(min)"=2405.14999999851, "timestamp"=timestamp(3493872130 s since 1904-01-01), "Magn Field(T)"=0.0}, {"temperature"=14.354, "lorentzian"={"A (VHz)"=0.0, "f (Hz)"=0.0, "G (Hz)"=0.0, "phi(rad)"=0.0, "Q"=0.0, "Norm  Ampl"=0.0, "bg (V)"=0.0+0.0i, "4corners"={"z (-pi/2)"=0.0+0.0i, "z(inf)"=0.0+0.0i, "z (pi/2)"=0.0+0.0i, "z center"=0.0+0.0i, "z(0)"=0.0+0.0i, "radius"=0.0}}, "timestamp(min)"=2406.4833333343267, "timestamp"=timestamp(3493872210 s since 1904-01-01), "Magn Field(T)"=0.0}, {"temperature"=14.354, "lorentzian"={"A (VHz)"=0.0, "f (Hz)"=0.0, "G (Hz)"=0.0, "phi(rad)"=0.0, "Q"=0.0, "Norm  Ampl"=0.0, "bg (V)"=0.0+0.0i, "4corners"={"z (-pi/2)"=0.0+0.0i, "z(inf)"=0.0+0.0i, "z (pi/2)"=0.0+0.0i, "z center"=0.0+0.0i, "z(0)"=0.0+0.0i, "radius"=0.0}}, "timestamp(min)"=2407.8000000044703, "timestamp"=timestamp(3493872289 s since 1904-01-01), "Magn Field(T)"=0.0}, {"temperature"=14.358, "lorentzian"={"A (VHz)"=0.0, "f (Hz)"=0.0, "G (Hz)"=0.0, "phi(rad)"=0.0, "Q"=0.0, "Norm  Ampl"=0.0, "bg (V)"=0.0+0.0i, "4corners"={"z (-pi/2)"=0.0+0.0i, "z(inf)"=0.0+0.0i, "z (pi/2)"=0.0+0.0i, "z center"=0.0+0.0i, "z(0)"=0.0+0.0i, "radius"=0.0}}, "timestamp(min)"=2409.1166666671634, "timestamp"=timestamp(3493872368 s since 1904-01-01), "Magn Field(T)"=0.0}, {"temperature"=14.357, "lorentzian"={"A (VHz)"=0.0, "f (Hz)"=0.0, "G (Hz)"=0.0, "phi(rad)"=0.0, "Q"=0.0, "Norm  Ampl"=0.0, "bg (V)"=0.0+0.0i, "4corners"={"z (-pi/2)"=0.0+0.0i, "z(inf)"=0.0+0.0i, "z (pi/2)"=0.0+0.0i, "z center"=0.0+0.0i, "z(0)"=0.0+0.0i, "radius"=0.0}}, "timestamp(min)"=2410.4500000029802, "timestamp"=timestamp(3493872448 s since 1904-01-01), "Magn Field(T)"=0.0}, {"temperature"=14.356, "lorentzian"={"A (VHz)"=0.0, "f (Hz)"=0.0, "G (Hz)"=0.0, "phi(rad)"=0.0, "Q"=0.0, "Norm  Ampl"=0.0, "bg (V)"=0.0+0.0i, "4corners"={"z (-pi/2)"=0.0+0.0i, "z(inf)"=0.0+0.0i, "z (pi/2)"=0.0+0.0i, "z center"=0.0+0.0i, "z(0)"=0.0+0.0i, "radius"=0.0}}, "timestamp(min)"=2411.7666666656733, "timestamp"=timestamp(3493872527 s since 1904-01-01), "Magn Field(T)"=0.0}, {"temperature"=14.356, "lorentzian"={"A (VHz)"=0.0, "f (Hz)"=0.0, "G (Hz)"=0.0, "phi(rad)"=0.0, "Q"=0.0, "Norm  Ampl"=0.0, "bg (V)"=0.0+0.0i, "4corners"={"z (-pi/2)"=0.0+0.0i, "z(inf)"=0.0+0.0i, "z (pi/2)"=0.0+0.0i, "z center"=0.0+0.0i, "z(0)"=0.0+0.0i, "radius"=0.0}}, "timestamp(min)"=2413.083333335817, "timestamp"=timestamp(3493872606 s since 1904-01-01), "Magn Field(T)"=0.0}, {"temperature"=14.354, "lorentzian"={"A (VHz)"=0.0, "f (Hz)"=0.0, "G (Hz)"=0.0, "phi(rad)"=0.0, "Q"=0.0, "Norm  Ampl"=0.0, "bg (V)"=0.0+0.0i, "4corners"={"z (-pi/2)"=0.0+0.0i, "z(inf)"=0.0+0.0i, "z (pi/2)"=0.0+0.0i, "z center"=0.0+0.0i, "z(0)"=0.0+0.0i, "radius"=0.0}}, "timestamp(min)"=2414.416666664183, "timestamp"=timestamp(3493872686 s since 1904-01-01), "Magn Field(T)"=0.0}, {"temperature"=14.35, "lorentzian"={"A (VHz)"=0.0, "f (Hz)"=0.0, "G (Hz)"=0.0, "phi(rad)"=0.0, "Q"=0.0, "Norm  Ampl"=0.0, "bg (V)"=0.0+0.0i, "4corners"={"z (-pi/2)"=0.0+0.0i, "z(inf)"=0.0+0.0i, "z (pi/2)"=0.0+0.0i, "z center"=0.0+0.0i, "z(0)"=0.0+0.0i, "radius"=0.0}}, "timestamp(min)"=2415.7333333343267, "timestamp"=timestamp(3493872765 s since 1904-01-01), "Magn Field(T)"=0.0}, {"temperature"=14.352, "lorentzian"={"A (VHz)"=0.0, "f (Hz)"=0.0, "G (Hz)"=0.0, "phi(rad)"=0.0, "Q"=0.0, "Norm  Ampl"=0.0, "bg (V)"=0.0+0.0i, "4corners"={"z (-pi/2)"=0.0+0.0i, "z(inf)"=0.0+0.0i, "z (pi/2)"=0.0+0.0i, "z center"=0.0+0.0i, "z(0)"=0.0+0.0i, "radius"=0.0}}, "timestamp(min)"=2417.0666666701436, "timestamp"=timestamp(3493872845 s since 1904-01-01), "Magn Field(T)"=0.0}, {"temperature"=14.354, "lorentzian"={"A (VHz)"=0.0, "f (Hz)"=0.0, "G (Hz)"=0.0, "phi(rad)"=0.0, "Q"=0.0, "Norm  Ampl"=0.0, "bg (V)"=0.0+0.0i, "4corners"={"z (-pi/2)"=0.0+0.0i, "z(inf)"=0.0+0.0i, "z (pi/2)"=0.0+0.0i, "z center"=0.0+0.0i, "z(0)"=0.0+0.0i, "radius"=0.0}}, "timestamp(min)"=2418.3833333328366, "timestamp"=timestamp(3493872924 s since 1904-01-01), "Magn Field(T)"=0.0}, {"temperature"=14.349, "lorentzian"={"A (VHz)"=0.0, "f (Hz)"=0.0, "G (Hz)"=0.0, "phi(rad)"=0.0, "Q"=0.0, "Norm  Ampl"=0.0, "bg (V)"=0.0+0.0i, "4corners"={"z (-pi/2)"=0.0+0.0i, "z(inf)"=0.0+0.0i, "z (pi/2)"=0.0+0.0i, "z center"=0.0+0.0i, "z(0)"=0.0+0.0i, "radius"=0.0}}, "timestamp(min)"=2419.7000000029802, "timestamp"=timestamp(3493873003 s since 1904-01-01), "Magn Field(T)"=0.0}, {"temperature"=14.349, "lorentzian"={"A (VHz)"=0.0, "f (Hz)"=0.0, "G (Hz)"=0.0, "phi(rad)"=0.0, "Q"=0.0, "Norm  Ampl"=0.0, "bg (V)"=0.0+0.0i, "4corners"={"z (-pi/2)"=0.0+0.0i, "z(inf)"=0.0+0.0i, "z (pi/2)"=0.0+0.0i, "z center"=0.0+0.0i, "z(0)"=0.0+0.0i, "radius"=0.0}}, "timestamp(min)"=2421.0333333313465, "timestamp"=timestamp(3493873083 s since 1904-01-01), "Magn Field(T)"=0.0}, {"temperature"=14.346, "lorentzian"={"A (VHz)"=0.0, "f (Hz)"=0.0, "G (Hz)"=0.0, "phi(rad)"=0.0, "Q"=0.0, "Norm  Ampl"=0.0, "bg (V)"=0.0+0.0i, "4corners"={"z (-pi/2)"=0.0+0.0i, "z(inf)"=0.0+0.0i, "z (pi/2)"=0.0+0.0i, "z center"=0.0+0.0i, "z(0)"=0.0+0.0i, "radius"=0.0}}, "timestamp(min)"=2422.35000000149, "timestamp"=timestamp(3493873162 s since 1904-01-01), "Magn Field(T)"=0.0}, {"temperature"=14.344, "lorentzian"={"A (VHz)"=0.0, "f (Hz)"=0.0, "G (Hz)"=0.0, "phi(rad)"=0.0, "Q"=0.0, "Norm  Ampl"=0.0, "bg (V)"=0.0+0.0i, "4corners"={"z 
